vi "request.vi"(0 "url":string, 3 "input cluster":T1) -> (6 "Output headers":string, 9 "Output Body":string)   [LabVIEW 2019]
uses:
  <vilib>/httpClient/POSTBuffer.vi
  <vilib>/httpClient/LabVIEWHTTPClient.lvlib
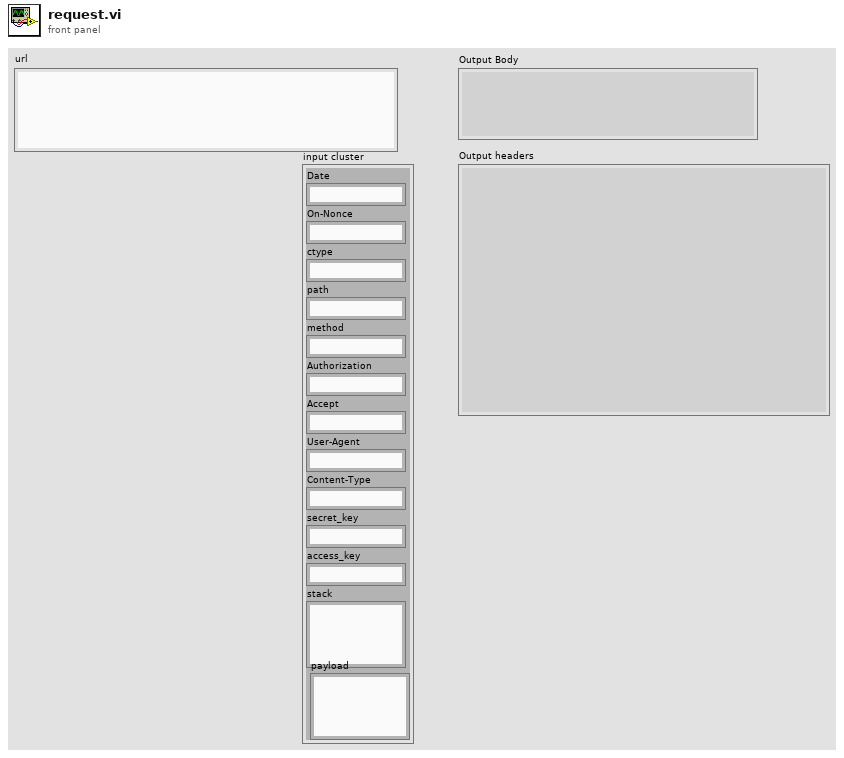
[diagram p1: front panel]
types:
  T1 = cluster{"Date":string, "On-Nonce":string, "ctype":string, "path":string, "method":string, "Authorization":string, "Accept":string, "User-Agent":string, "Content-Type":string, "secret_key":string, "access_key":string, "stack":string, "payload":string}
  T2 = typedef "LabVIEWHTTPClient.lvlib/ClientHandle.ctl" = refnum<k1>
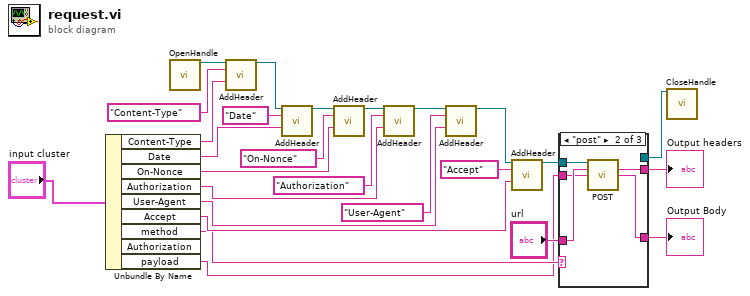
[diagram p0: block diagram]
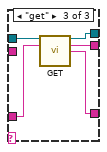
[diagram p3: hidden frame]
diagram:
  n1 = Unbundle By Name("input cluster") -> ("Content-Type"=w17:string, "Date"=w16:string, "On-Nonce"=w15:string, "Authorization"=w9:string, "User-Agent"=w14:string, "Accept"=w10:string, "method"=w8:string, "payload"=w1:string)  [unwired: 1 out]
  n2 = call <vilib>:"OpenHandle.vi"() -> ("client handle out"=w12:T2)  [unwired: 14 in, 1 out]
  n3 = call <vilib>:"AddHeader.vi"("client handle"=w12, "header"="Content-Type", "value"=w17) -> ("client handle out"=w26:T2)  [unwired: 11 in, 1 out]
  n4 = call <vilib>:"AddHeader.vi"("client handle"=w26, "header"="Date", "value"=w16) -> ("client handle out"=w25:T2)  [unwired: 11 in, 1 out]
  n5 = call <vilib>:"AddHeader.vi"("client handle"=w25, "header"="On-Nonce", "value"=w15) -> ("client handle out"=w24:T2)  [unwired: 11 in, 1 out]
  n6 = call <vilib>:"AddHeader.vi"("client handle"=w24, "header"="Authorization", "value"=w9) -> ("client handle out"=w23:T2)  [unwired: 11 in, 1 out]
  n7 = call <vilib>:"AddHeader.vi"("client handle"=w23, "header"="User-Agent", "value"=w14) -> ("client handle out"=w13:T2)  [unwired: 11 in, 1 out]
  n8 = call <vilib>:"AddHeader.vi"("client handle"=w13, "header"="Accept", "value"=w10) -> ("client handle out"=w7:T2)  [unwired: 11 in, 1 out]
  n9 = case shown="\"post\"" w8 {
    tunnel: w7 -> [_ w31 w36]
    tunnel: "url" -> [_ w30 w35]
    tunnel: [_ _ w34] -> w6
    tunnel: [_ w29 w32] -> w4
    tunnel: [_ w28 w33] -> w3
    tunnel: w1 -> [_ w27 _]
    frame "False", Default {
    }
    frame "post" {
      n10 = call-poly <vilib>:"POST.vi"("client handle"=w31, "url"=w30, "buffer"=w27) -> ("headers"=w28:string, "body"=w29:string)  [unwired: 9 in, 2 out]
    }
    frame "get" {
      n11 = call <vilib>:"GET.vi"("client handle"=w36, "url"=w35) -> ("client handle out"=w34:T2, "headers"=w33:string, "body"=w32:string)  [unwired: 10 in, 1 out]
    }
  }
  "Output Body" <- w4
  "Output headers" <- w3
  n12 = call <vilib>:"CloseHandle.vi"("client handle"=w6) -> ()  [unwired: 14 in, 1 out]
